vi "Autonomous.vi"   [LabVIEW 2020]
doc: "This VI starts when autonomous period begins, and will automatically be terminated when it ends. You can carry out timed or sensor driven operations directly to I/O or to subsystems without needing to return to the caller."
uses:
  <vilib>/Rock Robotics/WPI/Utilities/WPI_GetSetVariantRefNum.vi
  <vilib>/Rock Robotics/Network Tables/NT Read String.vi
  Framework/Robot Global Data.vi
types:
  T1 = typedef "WPI_JoystickDevRef.ctl" = cluster{"Device":T2}
  T2 = typedef "WPI_JoystickDeviceEnum.ctl" = enum16{"USB 0", "USB 1", "USB 2", "USB 3", "USB 4", "USB 5"}
  T3 = typedef "Command Status Info.ctl" = cluster{"Name":string, "Status":T4, "notifier out":T5}
  T4 = typedef "Completion Status.ctl" = enum16{"Successful", "Aborted", "Incomplete"}
  T5 = typedef "Completion Notifier.ctl" = refnum<notifier>
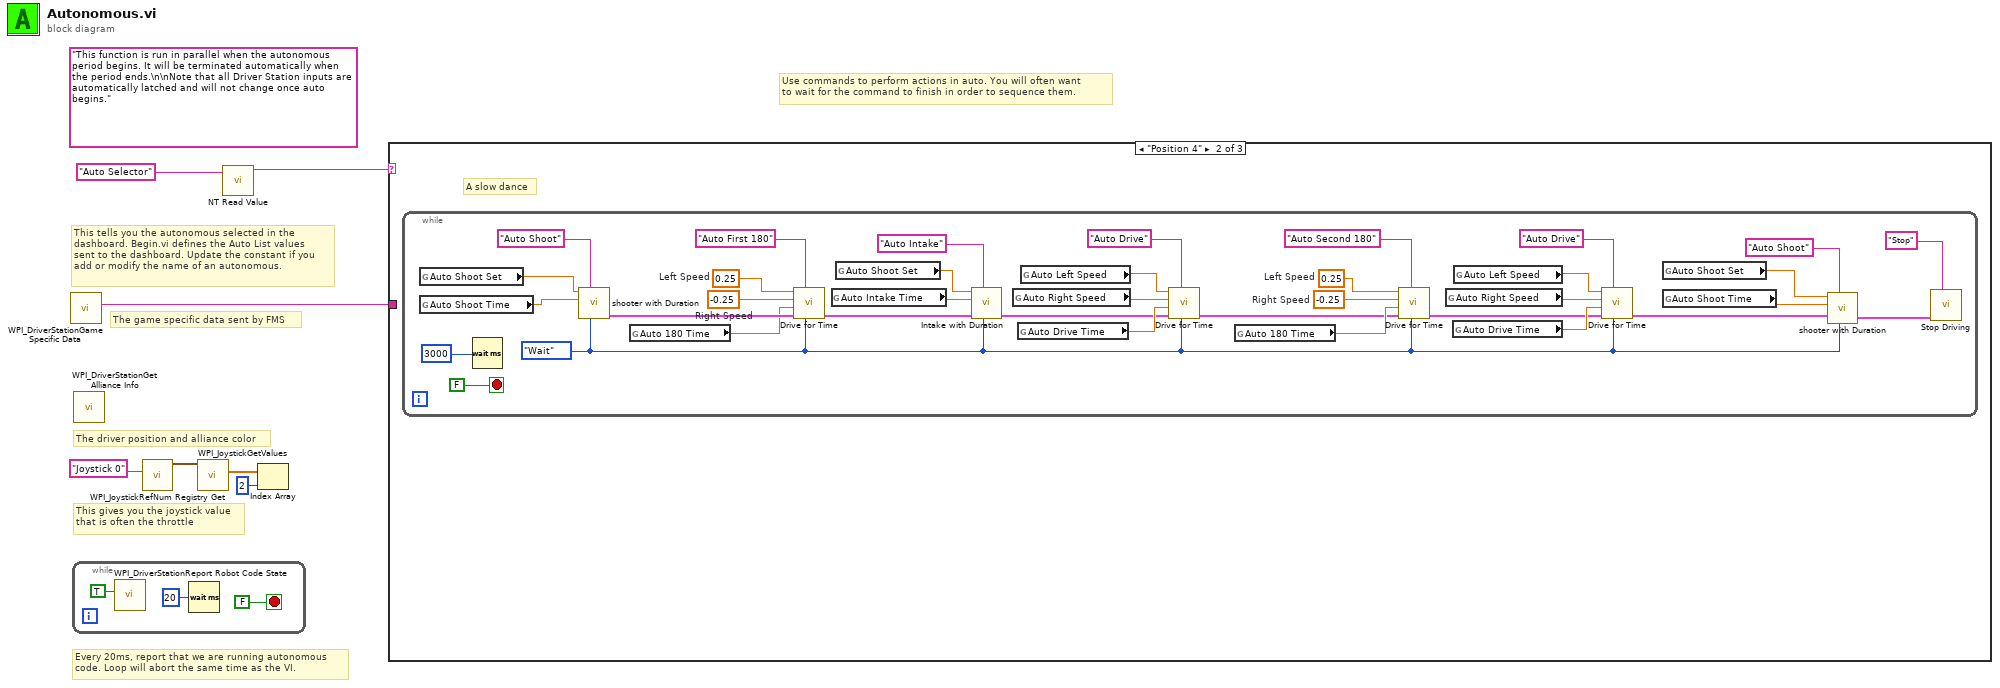
[diagram p0: block diagram]
diagram:
  (unwired) "This function is run in parallel when the autonomous period begins. It will be terminated automatically when the period ends.\n\nNote that all Driver Station inputs are automatically latched and will not change once auto begins."
  # "The game specific data sent by FMS"
  # "This tells you the autonomous selected in the \ndashboard. Begin.vi defines the Auto List values\nsent to the dashboard. Update the constant if you\nadd or modify the name of an autonomous."
  # "Every 20ms, report that we are running autonomous\ncode. Loop will abort the same time as the VI."
  # "This gives you the joystick value\nthat is often the throttle"
  # "Use commands to perform actions in auto. You will often want\nto wait for the command to finish in order to sequence them."
  # "The driver position and alliance color"
  n1 = call <vilib>:"WPI_DriverStationGame Specific Data.vi"() -> ("Game Specific Data"=w1:string)  [unwired: 11 in]
  n2 = while {
    stop <- FALSE stop-if-true
    n3 = call <vilib>:"WPI_DriverStationReport Robot Code State.vi"("Autonomous"=TRUE) -> ()  [unwired: 10 in, 1 out]
    n4 = Wait (ms)(milliseconds to wait=u32 20) -> ()  [unwired: 1 out]
  }
  n5 = call <vilib>:"WPI_DriverStationGet Alliance Info.vi"() -> ()  [unwired: 12 out]
  n6 = call <vilib>:"WPI_JoystickRefNum Registry Get.vi"("refnum name"="Joystick 0") -> ("JoystickDevRef"=w6:T1)  [unwired: 1 in, 9 out]
  n7 = call <vilib>:"WPI_JoystickGetValues.vi"("JoystickDevRef"=w6) -> ("Axes"=w5:dbl[])  [unwired: 6 in, 4 out]
  n8 = call-poly <vilib>:"NT Read Value.vi"("Name"="Auto Selector") -> ("String"=w2:string)  [unwired: 9 in, 1 out]
  n9 = Index Array(array=w5, index=2) -> ()  [unwired: 1 out]
  n10 = case shown="\"Position 4\"" w2 {
    tunnel: w1 -> [_ _ _]
    frame Default {
      # "You can put your main auto here, or you can right-click on the case and make any\nother frame be the default case."
      # "This is the frame that will execute if no selection is made, or if it is not recognized"
    }
    frame "Position 4" {
      # "A slow dance"
      n11 = while {
        stop <- FALSE stop-if-true
        w15 = -0.25  # Right Speed
        w14 = 0.25  # Left Speed
        w20 = -0.25  # Right Speed
        w21 = 0.25  # Left Speed
        w11 = enum16{"Start", "Wait"}."Wait" ("Synchronication")
        n12 = global read "Robot Global Data.vi" "Auto Shoot Set"() -> (w42:dbl)
        n13 = global read "Robot Global Data.vi" "Auto Shoot Time"() -> (w41:dbl)
        n14 = Wait (ms)(milliseconds to wait=u32 3000 ("millisecond timer value")) -> ()  [unwired: 1 out]
        n15 = call "shooter with Duration .vi"("Synchronization"=w11, "Description"="Auto Shoot", "Duration (s)"=w41, "Setpoint"=w42) -> ("Command Info Out"=w22:T3)  [unwired: 7 in]
        n16 = global read "Robot Global Data.vi" "Auto 180 Time"() -> (w19:dbl)
        n17 = call "Drive for Time.vi"("Synchronization"=w11, "Description"="Auto First 180", "Command Info In"=w22, "Seconds"=w19, "Right Speed"=w20, "Left Speed"=w21) -> ("Command Info Out"=w23:T3)  [unwired: 5 in]
        n18 = global read "Robot Global Data.vi" "Auto Intake Time"() -> (w40:dbl)
        n19 = global read "Robot Global Data.vi" "Auto Shoot Set"() -> (w39:dbl)
        n20 = call "Intake with Duration .vi"("Synchronization"=w11, "Description"="Auto Intake", "Command Info In"=w23, "Duration (s)"=w40, "Setpoint"=w39) -> ("Command Info Out"=w30:T3)  [unwired: 6 in]
        n21 = global read "Robot Global Data.vi" "Auto Right Speed"() -> (w32:dbl)
        n22 = global read "Robot Global Data.vi" "Auto Drive Time"() -> (w31:dbl)
        n23 = global read "Robot Global Data.vi" "Auto Left Speed"() -> (w33:dbl)
        n24 = call "Drive for Time.vi"("Synchronization"=w11, "Description"="Auto Drive", "Command Info In"=w30, "Seconds"=w31, "Right Speed"=w32, "Left Speed"=w33) -> ("Command Info Out"=w13:T3)  [unwired: 5 in]
        n25 = global read "Robot Global Data.vi" "Auto 180 Time"() -> (w17:dbl)
        n26 = call "Drive for Time.vi"("Synchronization"=w11, "Description"="Auto Second 180", "Command Info In"=w13, "Seconds"=w17, "Right Speed"=w15, "Left Speed"=w14) -> ("Command Info Out"=w12:T3)  [unwired: 5 in]
        n27 = global read "Robot Global Data.vi" "Auto Right Speed"() -> (w36:dbl)
        n28 = global read "Robot Global Data.vi" "Auto Drive Time"() -> (w35:dbl)
        n29 = global read "Robot Global Data.vi" "Auto Left Speed"() -> (w37:dbl)
        n30 = call "Drive for Time.vi"("Synchronization"=w11, "Description"="Auto Drive", "Command Info In"=w12, "Seconds"=w35, "Right Speed"=w36, "Left Speed"=w37) -> ("Command Info Out"=w24:T3)  [unwired: 5 in]
        n31 = global read "Robot Global Data.vi" "Auto Shoot Set"() -> (w28:dbl)
        n32 = global read "Robot Global Data.vi" "Auto Shoot Time"() -> (w27:dbl)
        n33 = call "shooter with Duration .vi"("Synchronization"=w11, "Description"="Auto Shoot", "Command Info In"=w24, "Duration (s)"=w27, "Setpoint"=w28) -> ("Command Info Out"=w25:T3)  [unwired: 6 in]
        n34 = call "Stop Driving.vi"("Description"="Stop", "Command Info In"=w25) -> ()  [unwired: 9 in, 1 out]
      }
    }
    frame "Your Turn" {
    }
  }
